vi "Generate waveform3channel.vi"(8 "error in (no error)":errorcluster, 11 "Galvo in":refnum<class "InVivo_ImagingModeSPIM.lvclass">) -> (0 "error out":errorcluster, 2 "Array":variant[](array[variant]), 3 "Galvo out":refnum<class "InVivo_ImagingModeSPIM.lvclass">)   [LabVIEW 2012, in "InVivo_ImagingModeSPIM.lvclass"]
uses:
  InVivo_ImagingModeSPIM.lvclass
  InVivo_ImagingModeSPIM.lvclass/InVivo_ImagingModeSPIM.ctl
  <vilib>/measure/NI_MABase.lvlib
panel:
  out "Mixed Signal Graph":T1(graph)
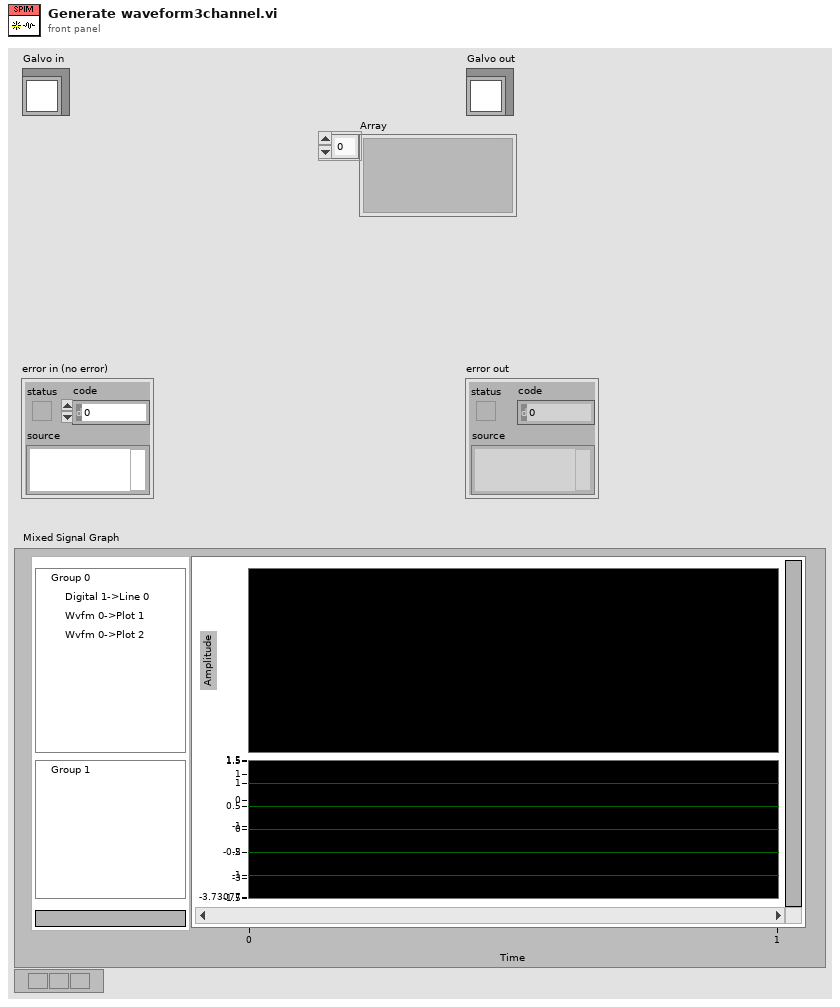
[diagram p1: front panel]
types:
  T1 = cluster{waveform(dbl)[], "digital waveform out":digitalwaveform}
  T2 = typedef "InVivo_ImagingModeSPIM.lvclass/waveform_enum.ctl" = enum16{"triangular", "sawtooth", "sinusodial"}
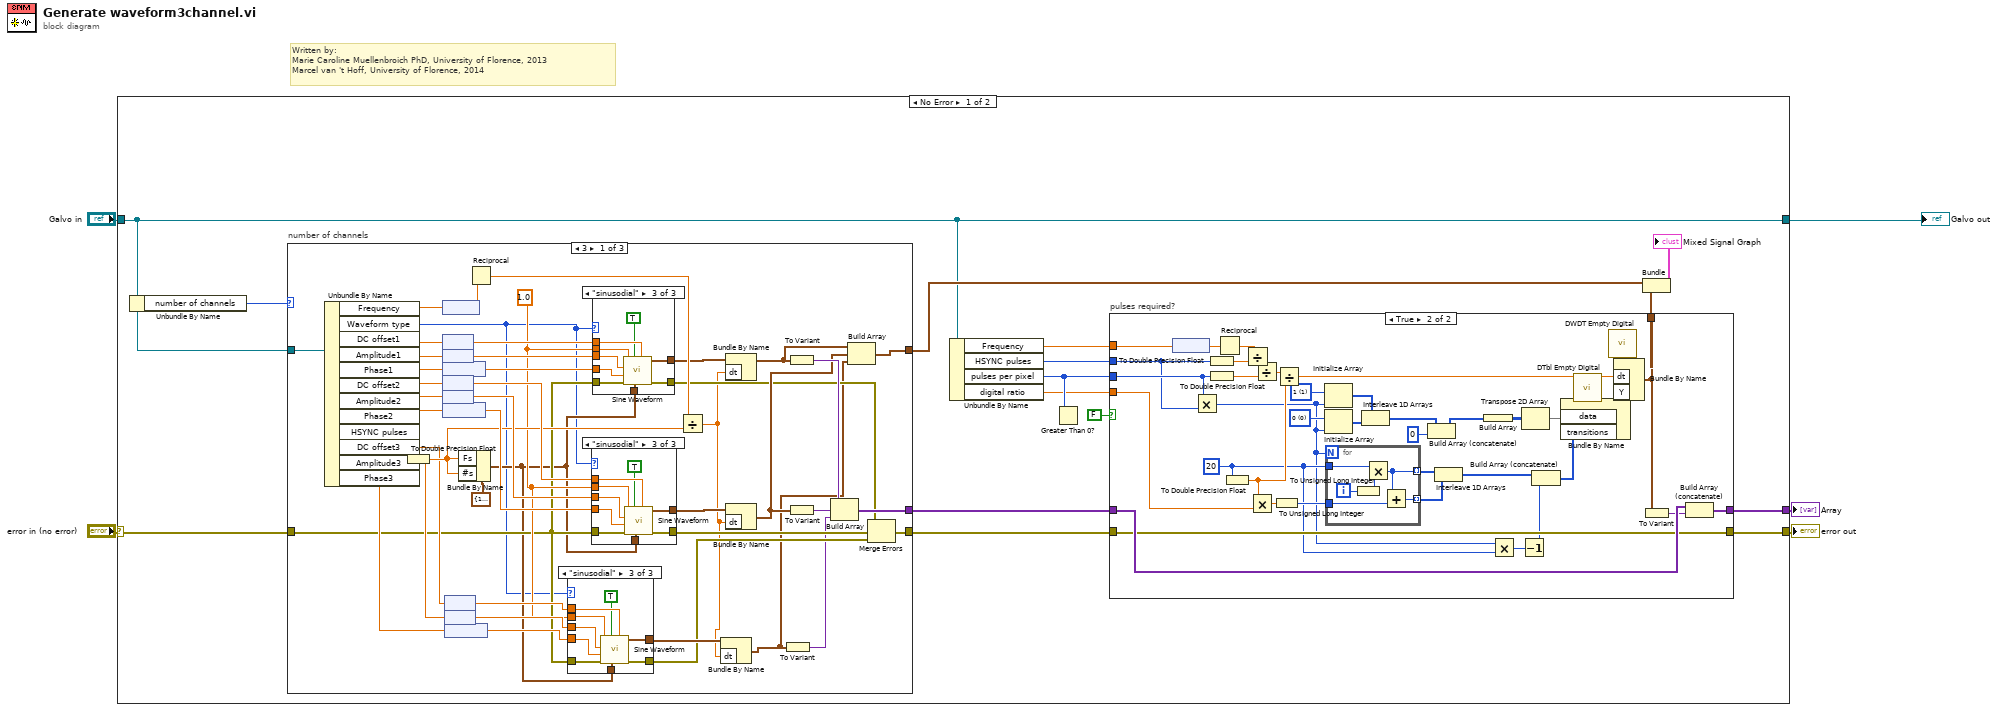
[diagram p0: block diagram]
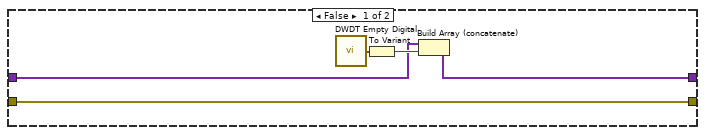
[diagram p2: hidden frame]
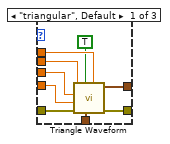
[diagram p3: hidden frame]
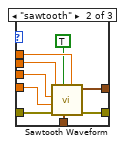
[diagram p4: hidden frame]
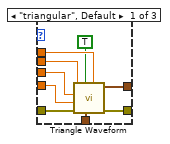
[diagram p5: hidden frame]
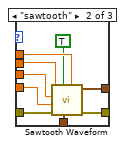
[diagram p6: hidden frame]
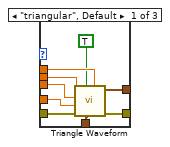
[diagram p7: hidden frame]
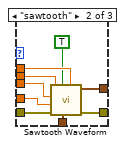
[diagram p8: hidden frame]
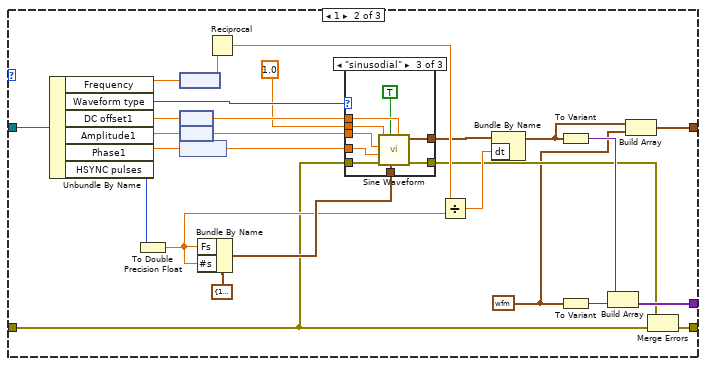
[diagram p9: hidden frame]
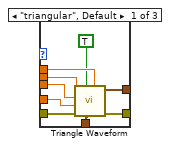
[diagram p10: hidden frame]
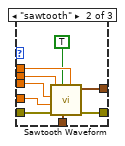
[diagram p11: hidden frame]
diagram:
  # "Written by:\nMarie Caroline Muellenbroich PhD, University of Florence, 2013 \nMarcel van 't Hoff, University of Florence, 2014"
  n1 = case shown="No Error" "error in (no error)" {
    selector: "error in (no error)" -> [w20 w253]
    tunnel: [w12 w253] -> w5
    tunnel: [w8 w252] -> w4
    tunnel: "Galvo in" -> [w8 w252]
    tunnel: [w18 _] -> w3
    frame No Error {
      n2 = Unbundle By Name(w8) -> ("number of channels"=w6:u8)
      n3 = case "number of channels" shown="3" w6 {
        tunnel: [w102 w214 w251] -> w19
        tunnel: w20 -> [w78 w199 w251]
        tunnel: [w101 w213 _] -> w17
        tunnel: [w89 w202 _] -> w10
        tunnel: w8 -> [w86 w197 _]
        frame 3 {
          w79 = 1.0
          n4 = Unbundle By Name(w86) -> ("Frequency"=w95:dbl[unit], "Waveform type"=w71:T2, "DC offset1"=w110:dbl[unit], "Amplitude1"=w111:dbl[unit], "Phase1"=w112:dbl[unit], "DC offset2"=w108:dbl[unit], "Amplitude2"=w107:dbl[unit], "Phase2"=w106:dbl[unit], "HSYNC pulses"=w105:i32, "DC offset3"=w85:dbl[unit], "Amplitude3"=w84:dbl[unit], "Phase3"=w83:dbl[unit])
          n5 = To Double Precision Float(number=w105) -> (double precision float=w93:dbl)
          n6 = node(w95) -> (w97:dbl)
          n7 = node(w110) -> (w114:dbl)
          n8 = node(w111) -> (w115:dbl)
          n9 = node(w112) -> (w94:dbl)
          n10 = node(w108) -> (w109:dbl)
          n11 = node(w107) -> (w103:dbl)
          n12 = node(w106) -> (w104:dbl)
          n13 = node(w85) -> (w82:dbl)
          n14 = node(w84) -> (w81:dbl)
          n15 = node(w83) -> (w80:dbl)
          n16 = Bundle By Name(cluster=cluster{"Fs":dbl, "#s":dbl} {"Fs"=1000.0, "#s"=1000.0} ("sampling info"), "Fs"=w93, "#s"=w93) -> (w77:cluster{"Fs":dbl, "#s":dbl})
          n17 = Reciprocal(x=w97) -> (1/x=w92:dbl)
          n18 = case shown="\"sinusodial\"" w71 {
            tunnel: w82 -> [w122 w133 w142]
            tunnel: w79 -> [w121 w132 w141]
            tunnel: w77 -> [w123 w131 w140]
            tunnel: [w120 w130 w139] -> w76
            tunnel: [w124 w125 w134] -> w75
            tunnel: w81 -> [w117 w128 w137]
            tunnel: w80 -> [w118 w127 w136]
            tunnel: w78 -> [w116 w126 w135]
            frame "triangular", Default {
              n19 = call <vilib>:"Triangle Waveform.vi"("offset"=w122, "sampling info"=w123, "reset signal"=TRUE, "error in (no error)"=w116, "phase"=w118, "amplitude"=w117, "frequency"=w121) -> ("error out"=w124:errorcluster, "signal out"=w120:waveform(dbl))  [unwired: 3 in]
            }
            frame "sawtooth" {
              n20 = call <vilib>:"Sawtooth Waveform.vi"("offset"=w133, "sampling info"=w131, "reset signal"=TRUE, "error in (no error)"=w126, "phase"=w127, "amplitude"=w128, "frequency"=w132) -> ("error out"=w125:errorcluster, "signal out"=w130:waveform(dbl))  [unwired: 3 in]
            }
            frame "sinusodial" {
              n21 = call <vilib>:"Sine Waveform.vi"("offset"=w142, "sampling info"=w140, "reset signal"=TRUE, "error in (no error)"=w135, "phase"=w136, "amplitude"=w137, "frequency"=w141) -> ("error out"=w134:errorcluster, "signal out"=w139:waveform(dbl))  [unwired: 3 in]
            }
          }
          n22 = case shown="\"sinusodial\"" w71 {
            tunnel: w109 -> [w149 w160 w169]
            tunnel: w79 -> [w148 w159 w168]
            tunnel: w77 -> [w150 w158 w167]
            tunnel: [w147 w157 w166] -> w96
            tunnel: [w151 w152 w161] -> w98
            tunnel: w103 -> [w144 w155 w164]
            tunnel: w104 -> [w145 w154 w163]
            tunnel: w78 -> [w143 w153 w162]
            frame "triangular", Default {
              n23 = call <vilib>:"Triangle Waveform.vi"("offset"=w149, "sampling info"=w150, "reset signal"=TRUE, "error in (no error)"=w143, "phase"=w145, "amplitude"=w144, "frequency"=w148) -> ("error out"=w151:errorcluster, "signal out"=w147:waveform(dbl))  [unwired: 3 in]
            }
            frame "sawtooth" {
              n24 = call <vilib>:"Sawtooth Waveform.vi"("offset"=w160, "sampling info"=w158, "reset signal"=TRUE, "error in (no error)"=w153, "phase"=w154, "amplitude"=w155, "frequency"=w159) -> ("error out"=w152:errorcluster, "signal out"=w157:waveform(dbl))  [unwired: 3 in]
            }
            frame "sinusodial" {
              n25 = call <vilib>:"Sine Waveform.vi"("offset"=w169, "sampling info"=w167, "reset signal"=TRUE, "error in (no error)"=w162, "phase"=w163, "amplitude"=w164, "frequency"=w168) -> ("error out"=w161:errorcluster, "signal out"=w166:waveform(dbl))  [unwired: 3 in]
            }
          }
          n26 = case shown="\"sinusodial\"" w71 {
            tunnel: w114 -> [w176 w187 w196]
            tunnel: w79 -> [w175 w186 w195]
            tunnel: w115 -> [w174 w185 w194]
            tunnel: w94 -> [w173 w184 w193]
            tunnel: w77 -> [w177 w183 w192]
            tunnel: [w172 w182 w191] -> w90
            tunnel: [w178 w181 w190] -> w87
            tunnel: w78 -> [w170 w179 w188]
            frame "triangular", Default {
              n27 = call <vilib>:"Triangle Waveform.vi"("offset"=w176, "sampling info"=w177, "reset signal"=TRUE, "error in (no error)"=w170, "phase"=w173, "amplitude"=w174, "frequency"=w175) -> ("error out"=w178:errorcluster, "signal out"=w172:waveform(dbl))  [unwired: 3 in]
            }
            frame "sawtooth" {
              n28 = call <vilib>:"Sawtooth Waveform.vi"("offset"=w187, "sampling info"=w183, "reset signal"=TRUE, "error in (no error)"=w179, "phase"=w184, "amplitude"=w185, "frequency"=w186) -> ("error out"=w181:errorcluster, "signal out"=w182:waveform(dbl))  [unwired: 3 in]
            }
            frame "sinusodial" {
              n29 = call <vilib>:"Sine Waveform.vi"("offset"=w196, "sampling info"=w192, "reset signal"=TRUE, "error in (no error)"=w188, "phase"=w193, "amplitude"=w194, "frequency"=w195) -> ("error out"=w190:errorcluster, "signal out"=w191:waveform(dbl))  [unwired: 3 in]
            }
          }
          n30 = Divide(x=w92, y=w93) -> (x/y=w74:dbl)
          n31 = Bundle By Name(cluster=w76, "dt"=w74) -> (w72:waveform(dbl))
          n32 = Bundle By Name(cluster=w90, "dt"=w74) -> (w88:waveform(dbl))
          n33 = Bundle By Name(cluster=w96, "dt"=w74) -> (w91:waveform(dbl))
          n34 = To Variant(anything=w72) -> (Variant=w73:variant)
          n35 = To Variant(anything=w88) -> (Variant=w99:variant)
          n36 = To Variant(anything=w91) -> (Variant=w100:variant)
          n37 = Build Array(w99, w100, w73) -> (w101:variant[])
          n38 = Build Array(w88, w91, w72) -> (w89:waveform(dbl)[])
          n39 = Merge Errors(w87, w98, w75) -> (w102:errorcluster)
        }
        frame 1 {
          w198 = waveform(dbl) {"t0"=timestamp(0 s since 1904-01-01), "dt"=1.0, "Y"=[]} ("signal out")
          n40 = Unbundle By Name(w197) -> ("Frequency"=w208:dbl[unit], "Waveform type"=w217:T2, "DC offset1"=w218:dbl[unit], "Amplitude1"=w219:dbl[unit], "Phase1"=w220:dbl[unit], "HSYNC pulses"=w216:i32)
          n41 = To Double Precision Float(number=w216) -> (double precision float=w206:dbl)
          n42 = node(w208) -> (w209:dbl)
          n43 = node(w218) -> (w222:dbl)
          n44 = node(w219) -> (w223:dbl)
          n45 = node(w220) -> (w207:dbl)
          n46 = Bundle By Name(cluster=cluster{"Fs":dbl, "#s":dbl} {"Fs"=1000.0, "#s"=1000.0} ("sampling info"), "Fs"=w206, "#s"=w206) -> (w215:cluster{"Fs":dbl, "#s":dbl})
          n47 = Reciprocal(x=w209) -> (1/x=w205:dbl)
          n48 = case shown="\"sinusodial\"" w217 {
            tunnel: w222 -> [w230 w241 w250]
            tunnel: 1.0 -> [w229 w240 w249]
            tunnel: w223 -> [w228 w239 w248]
            tunnel: w207 -> [w227 w238 w247]
            tunnel: w215 -> [w231 w237 w246]
            tunnel: [w226 w236 w245] -> w203
            tunnel: [w232 w235 w244] -> w200
            tunnel: w199 -> [w224 w233 w242]
            frame "triangular", Default {
              n49 = call <vilib>:"Triangle Waveform.vi"("offset"=w230, "sampling info"=w231, "reset signal"=TRUE, "error in (no error)"=w224, "phase"=w227, "amplitude"=w228, "frequency"=w229) -> ("error out"=w232:errorcluster, "signal out"=w226:waveform(dbl))  [unwired: 3 in]
            }
            frame "sawtooth" {
              n50 = call <vilib>:"Sawtooth Waveform.vi"("offset"=w241, "sampling info"=w237, "reset signal"=TRUE, "error in (no error)"=w233, "phase"=w238, "amplitude"=w239, "frequency"=w240) -> ("error out"=w235:errorcluster, "signal out"=w236:waveform(dbl))  [unwired: 3 in]
            }
            frame "sinusodial" {
              n51 = call <vilib>:"Sine Waveform.vi"("offset"=w250, "sampling info"=w246, "reset signal"=TRUE, "error in (no error)"=w242, "phase"=w247, "amplitude"=w248, "frequency"=w249) -> ("error out"=w244:errorcluster, "signal out"=w245:waveform(dbl))  [unwired: 3 in]
            }
          }
          n52 = Divide(x=w205, y=w206) -> (x/y=w204:dbl)
          n53 = Bundle By Name(cluster=w203, "dt"=w204) -> (w201:waveform(dbl))
          n54 = To Variant(anything=w201) -> (Variant=w211:variant)
          n55 = To Variant(anything=w198) -> (Variant=w212:variant)
          n56 = Build Array(w211, w212) -> (w213:variant[])
          n57 = Build Array(w201, w198) -> (w202:waveform(dbl)[])
          n58 = Merge Errors(w200, w199) -> (w214:errorcluster)
        }
        frame Default {
        }
      }
      n59 = Unbundle By Name(w8) -> ("Frequency"=w16:dbl[unit], "HSYNC pulses"=w15:i32, "pulses per pixel"=w13:i32, "digital ratio"=w11:dbl)
      n60 = Greater Than 0?(x=w13) -> ()  [unwired: 1 out]
      n61 = case "pulses required?" shown="True" FALSE {
        tunnel: w13 -> [_ w29]
        tunnel: [w25 w46] -> w12
        tunnel: w19 -> [w25 w46]
        tunnel: [w21 w59] -> w18
        tunnel: w17 -> [w22 w60]
        tunnel: w16 -> [_ w64]
        tunnel: w15 -> [_ w26]
        tunnel: [_ w56] -> w9
        tunnel: w11 -> [_ w42]
        frame False {
          n62 = call <vilib>:"DWDT Empty Digital.vi"() -> ("digital waveform out"=w23:digitalwaveform)  [unwired: 5 in]
          n63 = To Variant(anything=w23) -> (Variant=w24:variant)
          n64 = Build Array (concatenate)(w22, w24) -> (w21:variant[])
        }
        frame True {
          w30 = u32 20 ("ratio step size")
          w48 = u8 0 items=["0", "1", "Z", "L", "H", "X", "T", "V"] ("value 2")
          w47 = u8 1 items=["0", "1", "Z", "L", "H", "X", "T", "V"] ("value 2")
          n65 = node(w64) -> (w63:dbl)
          n66 = Multiply(x=w29, y=w26) -> (x*y=w27:i32)
          n67 = To Double Precision Float(number=w26) -> (double precision float=w61:dbl)
          n68 = To Double Precision Float(number=w29) -> (double precision float=w57:dbl)
          n69 = Reciprocal(x=w63) -> (1/x=w62:dbl)
          n70 = To Double Precision Float(number=w30) -> (double precision float=w41:dbl)
          n71 = Divide(x=w62, y=w61) -> (x/y=w58:dbl)
          n72 = Multiply(x=w41, y=w42) -> (x*y=w52:dbl)
          n73 = Divide(x=w58, y=w57) -> (x/y=w40:dbl)
          n74 = To Unsigned Long Integer(number=w52) -> (unsigned 32bit integer=w55:u32)
          n75 = Divide(x=w40, y=w41) -> (x/y=w39:dbl)
          n76 = Initialize Array(w47, w27) -> (w50:u8[])
          n77 = Initialize Array(w48, w27) -> (w51:u8[])
          n78 = for {
            N: w27 -> [_]
            tunnel: w55 -> [w68]
            tunnel: w30 -> [w70]
            tunnel: [w67] -> w53 mode=indexing
            tunnel: [w66] -> w54 mode=indexing
            i -> [w69]
            n79 = To Unsigned Long Integer(number=w69) -> (unsigned 32bit integer=w65:u32)
            n80 = Multiply(x=w70, y=w65) -> (x*y=w67:u32)
            n81 = Add(x=w67, y=w68) -> (x+y=w66:u32)
          }
          n82 = Interleave 1D Arrays(w50, w51) -> (w35:u8[])
          n83 = Build Array (concatenate)(w35, u8 0 ("value 2")) -> (w34:u8[])
          n84 = Interleave 1D Arrays(w53, w54) -> (w33:u32[])
          n85 = Build Array(w34) -> (w49:u8[][])
          n86 = Multiply(x=w27, y=w30) -> (x*y=w31:u32)
          n87 = Decrement(x=w31) -> (x-1=w28:u32)
          n88 = Transpose 2D Array(2D array=w49) -> (transposed array=w37:u8[][])
          n89 = Build Array (concatenate)(w33, w28) -> (w32:u32[])
          n90 = call <vilib>:"DTbl Empty Digital.vi"() -> ("digital data"=w45:digitaldata)  [unwired: 5 in]
          n91 = Bundle By Name(cluster=w45, "data"=w37, "transitions"=w32) -> (w43:digitaldata)
          n92 = call <vilib>:"DWDT Empty Digital.vi"() -> ("digital waveform out"=w44:digitalwaveform)  [unwired: 5 in]
          n93 = Bundle By Name(cluster=w44, "dt"=w39, "Y"=w43) -> (w56:digitalwaveform)
          n94 = To Variant(anything=w56) -> (Variant=w38:variant)
          n95 = Build Array (concatenate)(w60, w38) -> (w59:variant[])
        }
      }
      n96 = Bundle(w10, "digital waveform out"=w9) -> (→"Mixed Signal Graph":T1)  [unwired: 1 in]
    }
    frame Error {
    }
  }
  "error out" <- w5
  "Galvo out" <- w4
  "Array" <- w3
